vi "Read Integer.vi"(8 "error in (no error)":errorcluster, 11 "KDemoDerived in":refnum<class "KDemoDerived.lvclass">) -> (0 "error out":errorcluster, 2 "Integer":i32, 3 "KDemoDerived out":refnum<class "KDemoDerived.lvclass">)   [LabVIEW 2015, in "KDemoDerived.lvclass"]
uses:
  KDemoDerived.lvclass
  KDemoDerived.lvclass/KDemoDerived.ctl
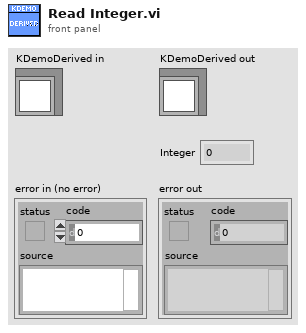
[diagram p1: front panel]
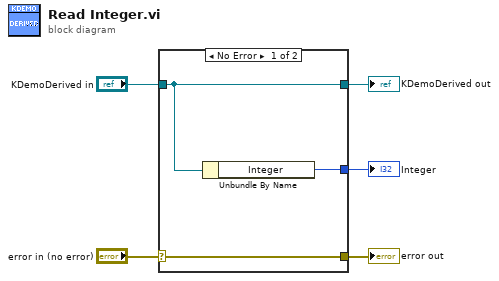
[diagram p0: block diagram]
diagram:
  n1 = case shown="No Error" "error in (no error)" {
    selector: "error in (no error)" -> [w8 w9]
    tunnel: [w8 w9] -> w4
    tunnel: [w7 w10] -> w2
    tunnel: "KDemoDerived in" -> [w7 w10]
    tunnel: [w6 _] -> w1
    frame No Error {
      n2 = Unbundle By Name(w7) -> ("Integer"=w6:i32)
    }
    frame Error {
    }
  }
  "error out" <- w4
  "KDemoDerived out" <- w2
  "Integer" <- w1
